vi "dialog_box for record.vi"(8 "错误输入（无错误）":errorcluster) -> (0 "错误输出":errorcluster, 2 "参数输出":T2, 3 "Cancelled?":bool caption="取消？", 6 "校准完毕？":bool)   [LabVIEW 2013]
doc: "该模板用于创建能够进行事件处理的对话框。"
uses:
  parameter set for record.ctl
panel:
  in  "测量终点":dbl
  in  "停留时间":dbl
  in  "总步数":dbl
  in  "步长":dbl
  in  "绷紧时间":dbl
  in  "松弛时间":dbl
  in  "绷紧点":dbl
  in  "松弛点":dbl
  in  "旋转速度":dbl
  in  "最终转数":dbl
  in  "初始转数":dbl
  in  "加载率":dbl
  in  "数据存放路径":path
  in  "测量起点":dbl
  in  "测量模式":T1(ring)
  in  "Cancel":bool caption="取消"
  in  "OK":bool caption="确定"
  in  "参数设置":T2
  # "force ramp"
  # "通用"
  # "force clamp"
  # "force jump"
  # "磁铁旋转"
  # "force ramp"
  # "通用"
  # "force clamp"
  # "force jump"
  # "磁铁旋转"
  # "force ramp"
  # "通用"
  # "force clamp"
  # "force jump"
  # "磁铁旋转"
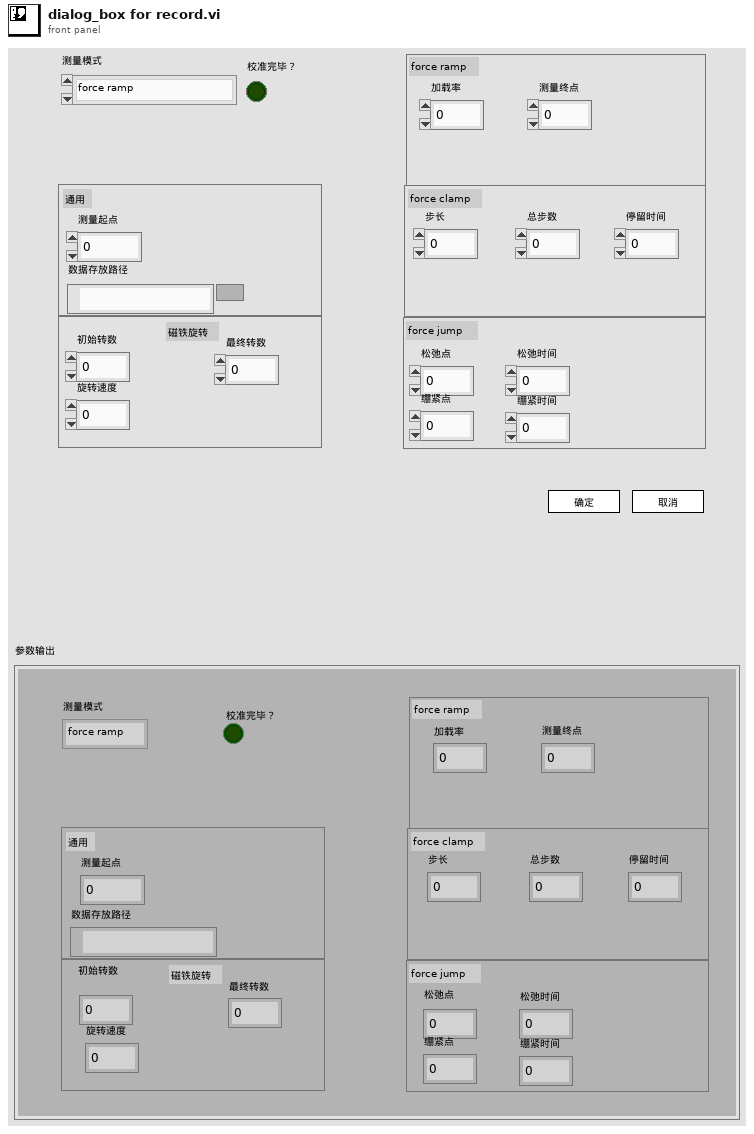
[diagram p1: front panel]
types:
  T1 = enum16{"force ramp", "force jump", "force clamp"}
  T2 = typedef "parameter set for record.ctl" = cluster{"测量模式":enum16{"force ramp", "force jump", "force clamp"}, "测量起点":dbl, "数据存放路径":path, "加载率":dbl, "初始转数":dbl, "最终转数":dbl, "旋转速度":dbl, "松弛点":dbl, "绷紧点":dbl, "松弛时间":dbl, "绷紧时间":dbl, "步长":dbl, "总步数":dbl, "停留时间":dbl, "测量终点":dbl, "校准完毕？":bool}
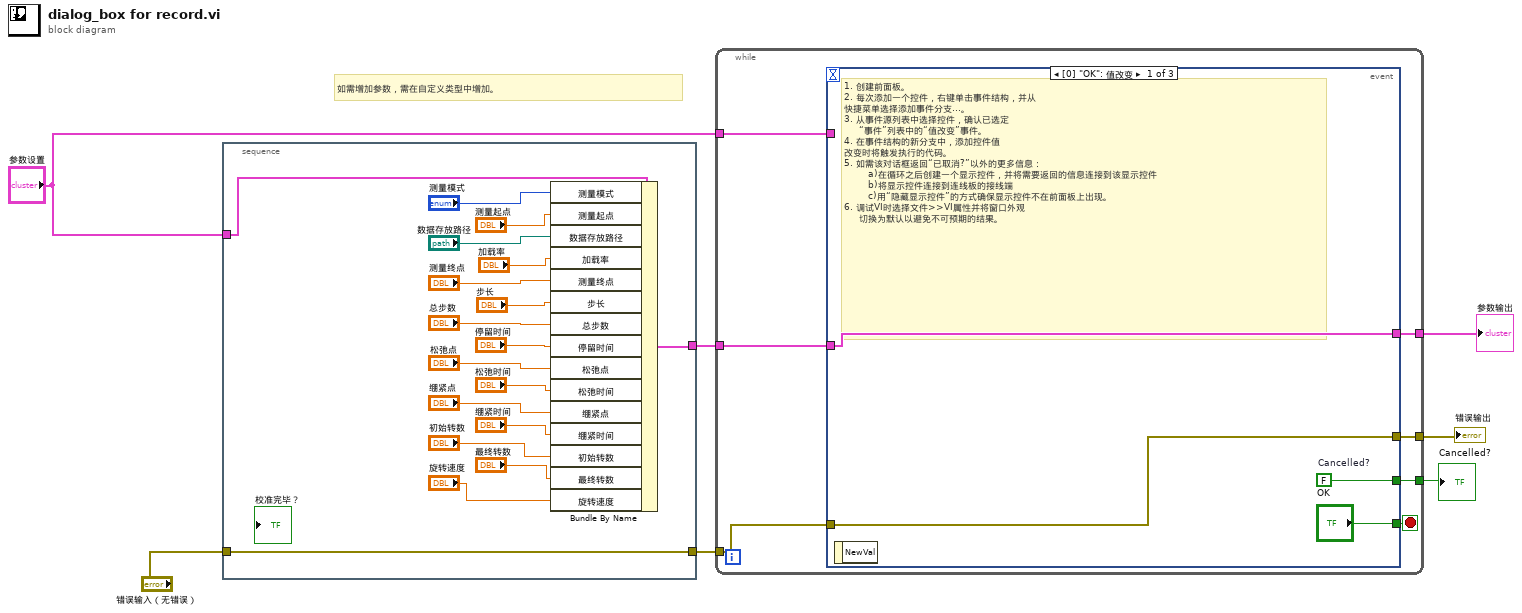
[diagram p0: block diagram]
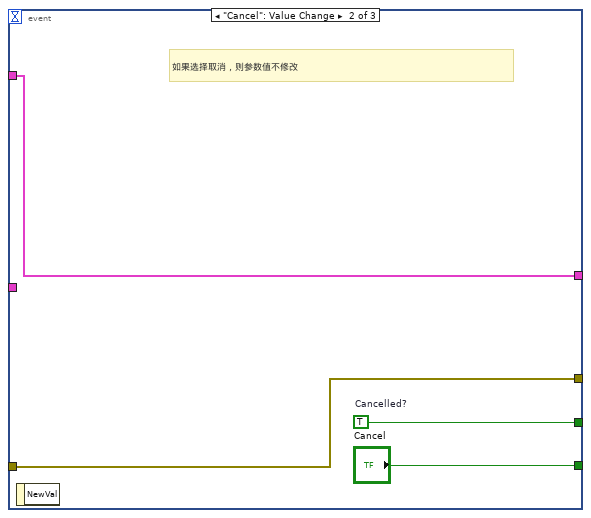
[diagram p2: hidden frame]
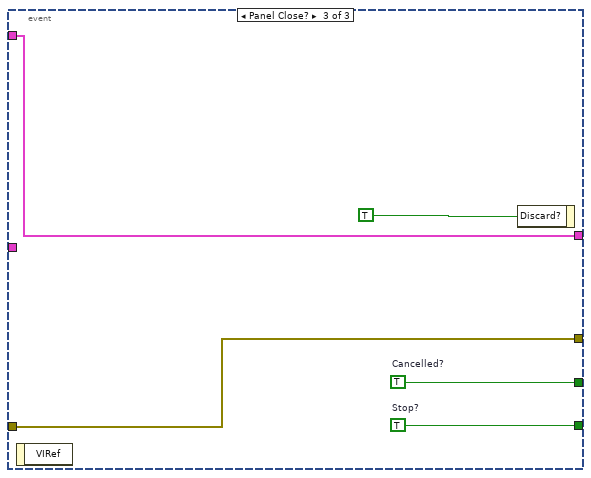
[diagram p3: hidden frame]
diagram:
  # "如需增加参数，需在自定义类型中增加。"
  n1 = stacked-sequence {
    tunnel: [w25] -> w6
    tunnel: "错误输入（无错误）" -> [w22]
    tunnel: [w22] -> w4
    tunnel: "参数设置" -> [w24]
    frame #0 {
      n2 = Bundle By Name(cluster=w24, "测量模式"="测量模式", "测量起点"="测量起点", "数据存放路径"="数据存放路径", "加载率"="加载率", "测量终点"="测量终点", "步长"="步长", "总步数"="总步数", "停留时间"="停留时间", "松弛点"="松弛点", "松弛时间"="松弛时间", "绷紧点"="绷紧点", "绷紧时间"="绷紧时间", "初始转数"="初始转数", "最终转数"="最终转数", "旋转速度"="旋转速度") -> (w25:T2)
    }
  }
  n3 = while {
    tunnel: [w31] -> w7
    tunnel: w6 -> [w30]
    tunnel: w4 -> [w29]
    tunnel: [w28] -> w3
    tunnel: [w27] -> w2
    tunnel: "参数设置" -> [w26]
    stop <- w32 stop-if-true
    n4 = event shown="[0] \"OK\": 值改变" {
      selector: _ -> [_ _ _]
      dyn-events: _ -> [_ _ _]
      timeout: _ -> [_ _ _]
      tunnel: ["OK" "Cancel" w44] -> w32
      tunnel: [w36 w40 w43] -> w31
      tunnel: w30 -> [w33 _ _]
      tunnel: [w34 w38 w42] -> w28
      tunnel: w29 -> [w34 w38 w42]
      tunnel: [w33 w37 w41] -> w27
      tunnel: w26 -> [_ w37 w41]
      event "OK": Value Change {
        w36 = FALSE  # Cancelled?
        # "1. 创建前面板。\n2. 每次添加一个控件，右键单击事件结构，并从\n快捷菜单选择添加事件分支...。\n3. 从事件源列表中选择控件，确认已选定\n     “事件”列表中的“值改变”事件。\n4. 在事件结构的新分支中，添加控件值\n改变时将触发执行的代码。\n5. 如需该对话框返回“已取消?”以外的更多信息：\n        a)在循环之后创建一个显示控件，并将需要返回的信息连接到该显示控件\n        b)将显示控件连接到连线板的接线端\n        c)用“隐藏显示控件”的方式确保显示控件不在前面板上出现。\n6. 调试VI时选择文件>>VI属性并将窗口外观\n     切换为默认以避免不可预期的结果。"
        n5 = event-data() -> ()  [unwired: 1 in, 1 out]
      }
      event "Cancel": Value Change {
        w40 = TRUE  # Cancelled?
        # "如果选择取消，则参数值不修改"
        n6 = event-data() -> ()  [unwired: 1 in, 1 out]
      }
      event Panel Close? {
        w43 = TRUE  # Cancelled?
        w44 = TRUE  # Stop?
        n7 = event-data() -> ()  [unwired: 1 in, 1 out]
        n8 = event-data("Discard?"=TRUE) -> ()  [unwired: 1 in, 1 out]
      }
    }
  }
  "Cancelled?" <- w7
  "错误输出" <- w3
  "参数输出" <- w2
